vi "Write ADU Packet.vi"(8 "error in":errorcluster, 9 "modbus data unit":refnum<class "Modbus Data Unit.lvclass">, 10 "protocol layer":refnum<class "Network Protocol.lvclass">, 11 "IP transmission data unit in":refnum<class "IP Data Unit.lvclass">) -> (0 "error out":errorcluster, 2 "protocol layer out":refnum<class "Network Protocol.lvclass">, 3 "IP transmission data unit out":refnum<class "IP Data Unit.lvclass">)   [LabVIEW 2012, in "IP Data Unit.lvclass"]
doc: "This uses the protocol layer to write a modbus packet to the bus, wrapped in the IP transmission data unit."
uses:
  IP Data Unit.lvclass
  Modbus Data Unit/Modbus Data Unit.lvclass
  Network Protocol/Network Protocol.lvclass
  Transmission Data Unit.lvclass/Transmission Data Unit.ctl
  Modbus Data Unit/Modbus Data Unit.lvclass/Modbus Data Unit.ctl
  IP Data Unit.lvclass/IP Data Unit.ctl
  Modbus Data Unit/Flatten PDU.vi
  Transmission Data Unit.lvclass
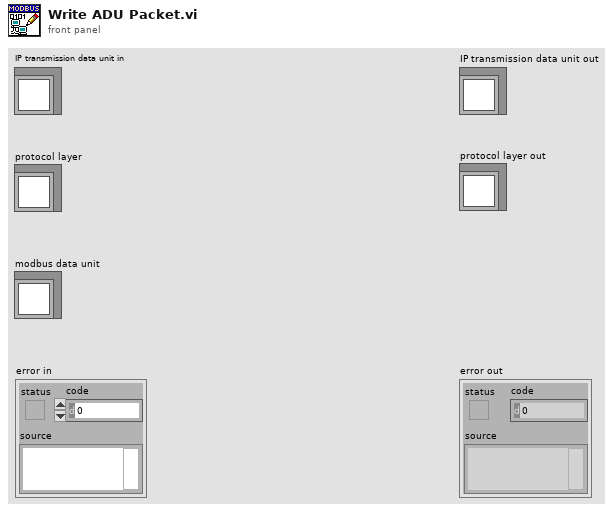
[diagram p1: front panel]
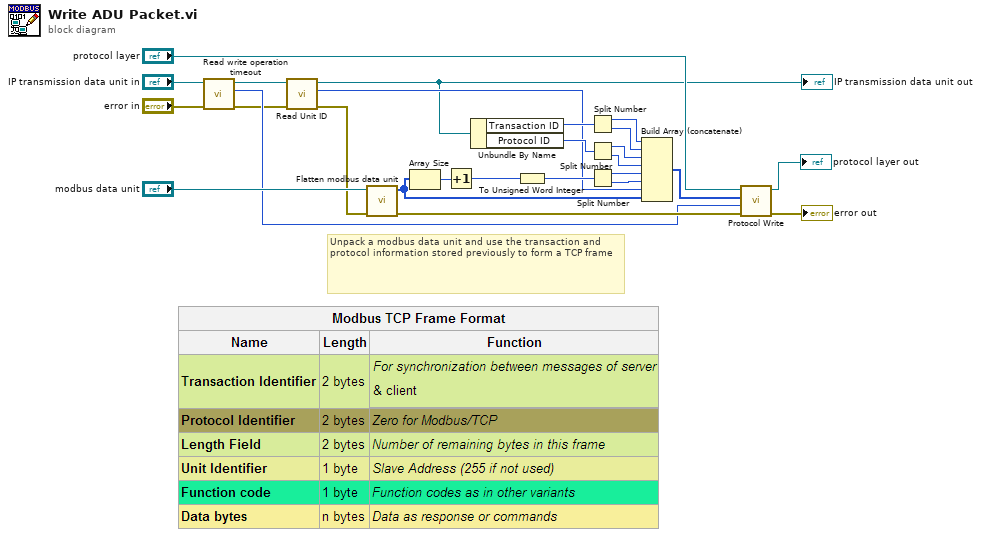
[diagram p0: block diagram]
diagram:
  # "Unpack a modbus data unit and use the transaction and protocol information stored previously to form a TCP frame"
  n1 = call "Read write operation timeout.vi"("error in (no error)"="error in", "transmission data unit in"="IP transmission data unit in") -> ("error out"=w6:errorcluster, "write operation timeout"=w7:i32, "transmission data unit out"=w5:refnum<class "IP Data Unit.lvclass">)  [unwired: 7 in]
  n2 = call "Read Unit ID.vi"("error in"=w6, "transmission data unit in"=w5) -> ("error out"=w2:errorcluster, "unit ID"=w8:u8, "transmission data unit out"=w1:refnum<class "IP Data Unit.lvclass">)  [unwired: 7 in]
  "IP transmission data unit out" <- w1
  n3 = call "Flatten modbus data unit.vi"("error in"=w2, "modbus data unit in"="modbus data unit") -> ("error out"=w10:errorcluster, "Full modbus data unit"=w9:u8[])  [unwired: 8 in]
  n4 = Array Size(array=w9) -> (size(s)=w22:i32)
  n5 = Increment(x=w22) -> (x+1=w19:i32)
  n6 = Unbundle By Name(w1) -> ("Transaction ID"=w21:u16, "Protocol ID"=w20:u16)
  n7 = To Unsigned Word Integer(number=w19) -> (unsigned 16bit integer=w18:u16)
  n8 = Split Number(x=w21) -> (hi(x)=w17:u8, lo(x)=w16:u8)
  n9 = Split Number(x=w20) -> (hi(x)=w15:u8, lo(x)=w14:u8)
  n10 = Split Number(x=w18) -> (hi(x)=w13:u8, lo(x)=w12:u8)
  n11 = Build Array (concatenate)(w17, w16, w15, w14, w13, w12, w8, w9) -> (w11:u8[])
  n12 = call-dynamic "Protocol Write.vi"("error in"=w10, "timeout"=w7, "data"=w11, "protocol layer in"="protocol layer") -> ("error out"=→"error out":errorcluster, "protocol layer out"=→"protocol layer out":refnum<class "Network Protocol.lvclass">)  [unwired: 5 in, 1 out]
